vi "onComputeNext.vi"(8 "error in (no error)":errorcluster, 9 "Time Stamp":timestamp, 10 "Expression":string, 11 "Cron.Quartz in":refnum<class "Cron.Quartz.lvclass">) -> (0 "error out":errorcluster, 1 "Next Occurence":timestamp, 3 "Cron.Quartz out":refnum<class "Cron.Quartz.lvclass">)   [LabVIEW 2013, in "openCron.lvlib" / "Cron.Quartz.lvclass"]
uses:
  Cron.Quartz.lvclass
panel:
  out "Array 2":T1(array[ring])
  out "Array":T2(array[cluster])
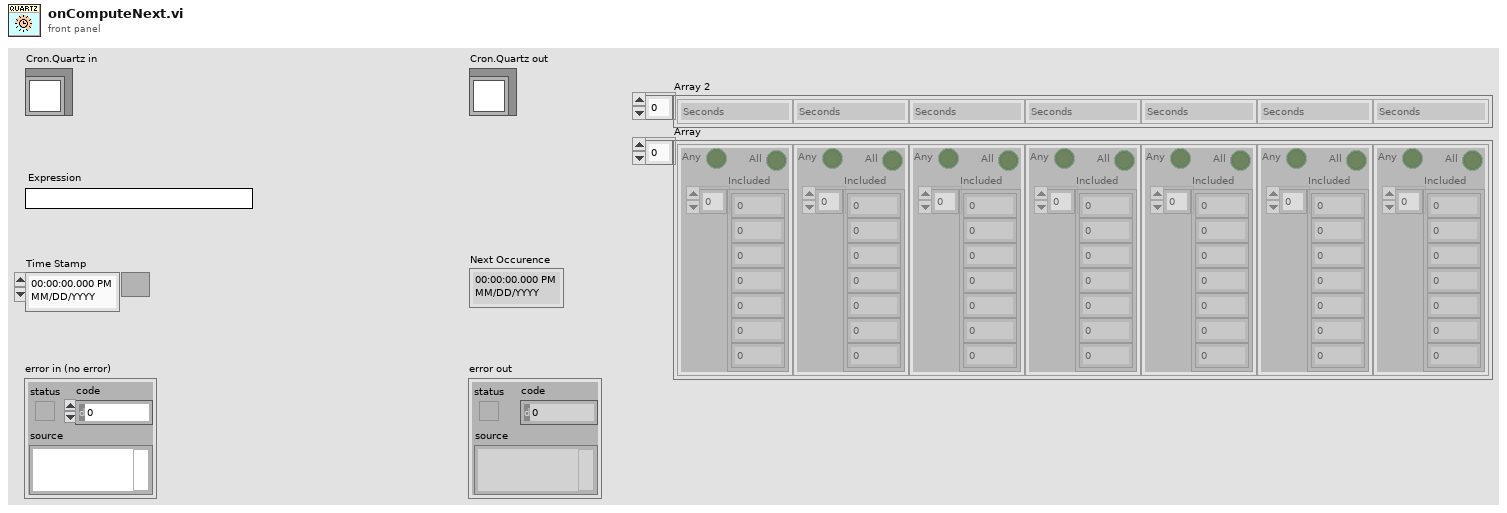
[diagram p1: front panel]
types:
  T1 = enum16{"Seconds", "Minutes", "Hours", "Day of Month", "Month", "Day of Week", "Year"}[]
  T2 = cluster{"Included":i32[], "All":bool, "Any":bool}[]
  T3 = cluster{"Included":i32[], "All":bool, "Any":bool}
  T4 = enum16{"Seconds", "Minutes", "Hours", "Day of Month", "Month", "Day of Week", "Year"}
  T5 = enum16{"SUN", "MON", "TUE", "WED", "THU", "FRI", "SAT"}
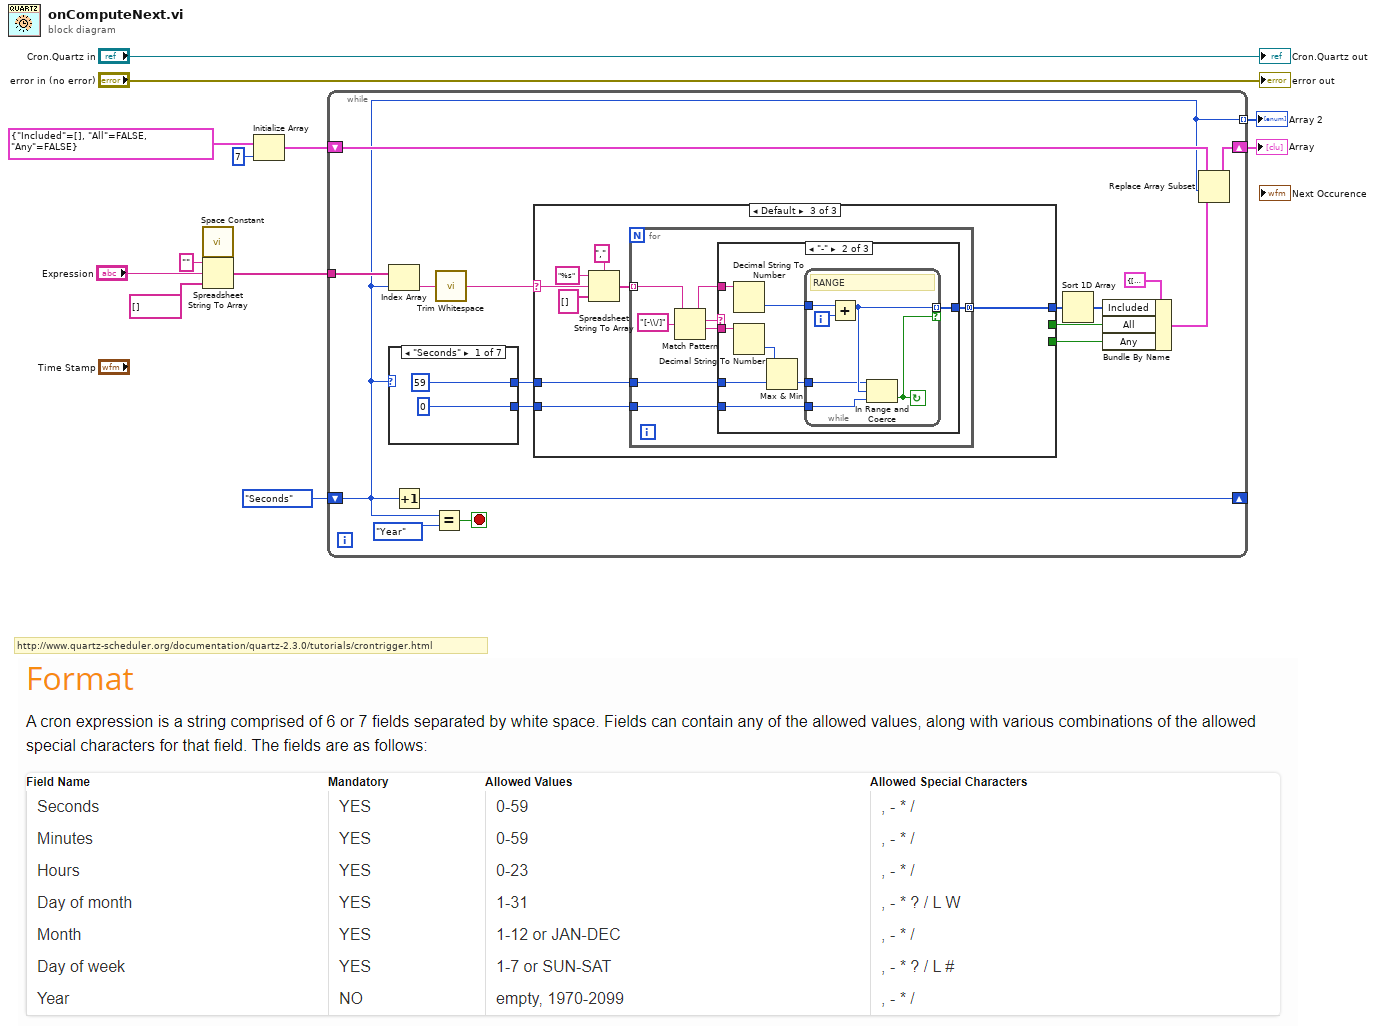
[diagram p0: block diagram]
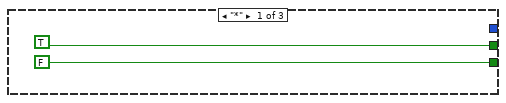
[diagram p2: hidden frame]
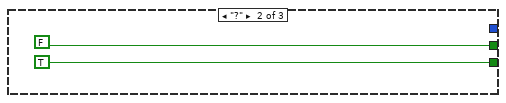
[diagram p3: hidden frame]
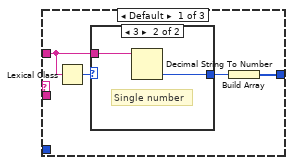
[diagram p4: hidden frame]
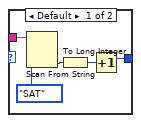
[diagram p5: hidden frame]
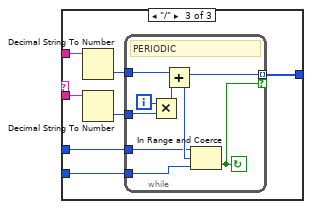
[diagram p6: hidden frame]
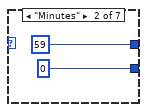
[diagram p7: hidden frame]
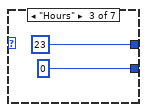
[diagram p8: hidden frame]
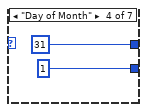
[diagram p9: hidden frame]
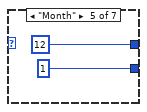
[diagram p10: hidden frame]
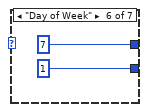
[diagram p11: hidden frame]
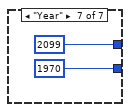
[diagram p12: hidden frame]
diagram:
  # "http://www.quartz-scheduler.org/documentation/quartz-2.3.0/tutorials/crontrigger.html"
  n1 = call <vilib>:"Space Constant.vi"() -> ("String"=w8:string)
  n2 = Spreadsheet String To Array(delimiter (Tab)=w8, format string="", spreadsheet string="Expression", array type (2D Dbl)=string[] []) -> (array=w7:string[])
  n3 = Initialize Array(T3 {"Included"=[], "All"=FALSE, "Any"=FALSE}, 7 ("dimension size")) -> (w3:T2)
  n4 = while {
    tunnel: w7 -> [w30]
    shift-right: [w27] -> _
    shift-left: T4."Seconds" -> [w14]
    shift-right: [w24] -> w2
    shift-left: w3 -> [w23]
    tunnel: [w14] -> w1 mode=indexing
    stop <- w28 stop-if-true
    n5 = Index Array(array=w30, index=w14) -> (element=w26:string)
    n6 = case shown="\"Seconds\"" w14 {
      tunnel: [59 ("y") 59 ("y") 23 ("y") 31 ("y") 12 ("y") 7 ("y") 2099 ("y")] -> w21
      tunnel: [0 ("y") 0 ("y") 0 ("y") 1 ("y") 1 ("y") 1 ("y") 1970 ("y")] -> w20
      frame "Seconds" {
      }
      frame "Minutes" {
      }
      frame "Hours" {
      }
      frame "Day of Month" {
      }
      frame "Month" {
      }
      frame "Day of Week" {
      }
      frame "Year" {
      }
    }
    n7 = Increment(x=w14) -> (x+1=w27:T4)
    n8 = Equal?(x=w14, y=T4."Year") -> (x = y?=w28:bool)
    n9 = call <vilib>:"Trim Whitespace.vi"("string"=w26) -> ("trimmed string"=w25:string)  [unwired: 1 in]
    n10 = case shown="Default" w25 {
      selector: w25 -> [_ _ w38]
      tunnel: [_ _ w37] -> w18
      tunnel: [TRUE FALSE _] -> w16
      tunnel: [FALSE TRUE _] -> w15
      tunnel: w21 -> [_ _ w36]
      tunnel: w20 -> [_ _ w35]
      frame "*" {
      }
      frame "?" {
      }
      frame Default {
        n11 = Spreadsheet String To Array(delimiter (Tab)=",", format string="%s", spreadsheet string=w38, array type (2D Dbl)=string[] []) -> (array=w39:string[])
        n12 = for {
          tunnel: w39 -> [w50] mode=indexing
          tunnel: [w46] -> w37 mode=concatenating
          tunnel: w36 -> [w44]
          tunnel: w35 -> [w43]
          n13 = Match Pattern(string=w50, regular expression="[-\\/]") -> (before substring=w47:string, match substring=w48:string, after substring=w45:string)  [unwired: 1 in, 1 out]
          n14 = case shown="\"-\"" w48 {
            tunnel: w47 -> [w52 w69 w82]
            tunnel: [w53 w66 w80] -> w46
            tunnel: w45 -> [_ w67 w78]
            tunnel: w44 -> [_ w64 w77]
            tunnel: w43 -> [_ w63 w76]
            frame Default {
              n15 = Lexical Class(1:w52) -> (0:w51:i16)
              n16 = case shown="3" w51 {
                tunnel: [w55 w61] -> w54
                tunnel: w52 -> [w59 w60]
                frame Default {
                  n17 = Scan From String(input string=w59, default 1=T5."SAT" ("y")) -> (output 1=w56:T5)  [unwired: 3 in, 3 out]
                  n18 = To Long Integer(number=w56) -> (32bit integer=w57:i32)
                  n19 = Increment(x=w57) -> (x+1=w55:i32)
                }
                frame 3 {
                  # "Single number"
                  n20 = Decimal String To Number(string=w60) -> (number=w61:i32)  [unwired: 2 in, 1 out]
                }
              }
              n21 = Build Array(w54) -> (w53:i32[])
            }
            frame "-" {
              n22 = Decimal String To Number(string=w69) -> (number=w68:i32)  [unwired: 2 in, 1 out]
              n23 = Decimal String To Number(string=w67) -> (number=w65:i32)  [unwired: 2 in, 1 out]
              n24 = Max & Min(x=w65, y=w64) -> (min(x,y)=w62:i32)  [unwired: 1 out]
              n25 = while {
                tunnel: w68 -> [w75]
                tunnel: [w72] -> w66 mode=indexing if=w73
                tunnel: w63 -> [w71]
                tunnel: w62 -> [w70]
                i -> [w74]
                stop <- w73 continue-if-true
                # "RANGE"
                n26 = Add(x=w75, y=w74) -> (x+y=w72:i32)
                n27 = In Range and Coerce(upper limit=w70, x=w72, lower limit=w71) -> (In Range?=w73:bool)  [unwired: 1 out]
              }
            }
            frame "/" {
              n28 = Decimal String To Number(string=w82) -> (number=w81:i32)  [unwired: 2 in, 1 out]
              n29 = Decimal String To Number(string=w78) -> (number=w79:i32)  [unwired: 2 in, 1 out]
              n30 = while {
                tunnel: w81 -> [w90]
                tunnel: [w86] -> w80 mode=indexing if=w83
                tunnel: w79 -> [w89]
                tunnel: w77 -> [w85]
                tunnel: w76 -> [w84]
                i -> [w88]
                stop <- w83 continue-if-true
                # "PERIODIC"
                n31 = Multiply(x=w88, y=w89) -> (x*y=w87:i32)
                n32 = Add(x=w90, y=w87) -> (x+y=w86:i32)
                n33 = In Range and Coerce(upper limit=w85, x=w86, lower limit=w84) -> (In Range?=w83:bool)  [unwired: 1 out]
              }
            }
          }
        }
      }
    }
    n34 = Sort 1D Array(array=w18) -> (sorted array=w19:i32[])
    n35 = Bundle By Name(cluster=T3 {"Included"=[], "All"=FALSE, "Any"=FALSE}, "Included"=w19, "All"=w16, "Any"=w15) -> (w22:T3)
    n36 = Replace Array Subset(array=w23, new element=w22, index=w14) -> (w24:T2)
  }
  "Array" <- w2
  "Array 2" <- w1
  "error out" <- "error in (no error)"
  "Cron.Quartz out" <- "Cron.Quartz in"
